vi "Spherical Bessel Function jn.vi"(2 "n":i32, 3 "x":dbl format="%.2f") -> (1 "jn(x)":dbl format="%.2f")   [LabVIEW 2020, in "NI_Gmath.lvlib"]
doc: "Calculates the spherical Bessel function of the first kind."
uses:
  <vilib>/gmath/NI_Gmath.lvlib
  <resource>/lvanlys.dll
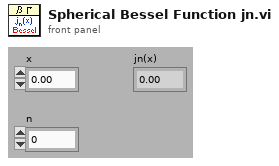
[diagram p1: front panel]
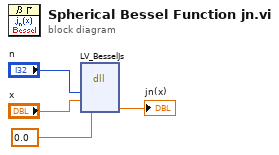
[diagram p0: block diagram]
diagram:
  n1 = dll-call lib="e:/builds/penguin/labview/branches/2020/dev/dist/resource/lvanlys.*" fn="LV_BesselJs"("n"="n", "x"="x", "jn(x)"=0.0 ("Jr")) -> ("jn(x)"=→"jn(x)":dbl)  [unwired: 6 in, 2 out]
